vi "Set Write Access.vi"(8 "error in (no error)":errorcluster, 10 "Write Access":enum8{"Allowed", "Required", "None"}(ring), 11 "abs_SharedVar_Bool in":refnum<class "conc_SharedVar_DBL.lvclass">) -> (0 "error out":errorcluster, 3 "abs_SharedVar_Bool out":refnum<class "conc_SharedVar_DBL.lvclass">)   [LabVIEW 2021, in "conc_SharedVar_DBL.lvclass"]
uses:
  conc_SharedVar_DBL.lvclass
  conc_SharedVar_DBL.lvclass/conc_SharedVar_DBL.ctl
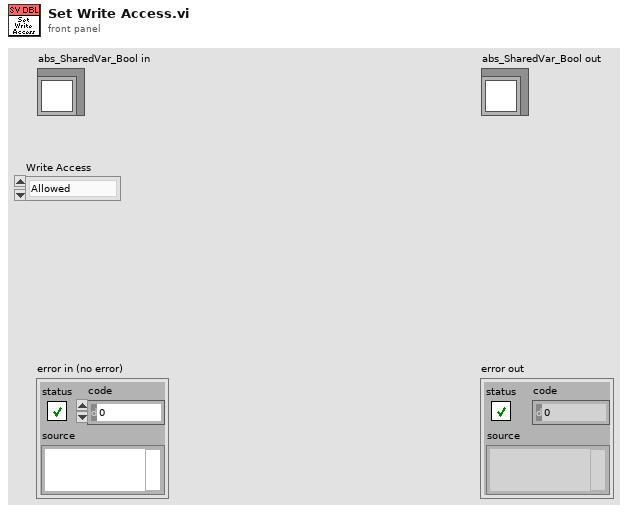
[diagram p1: front panel]
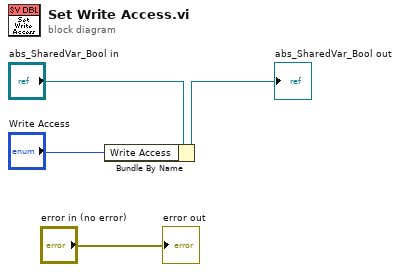
[diagram p0: block diagram]
diagram:
  n1 = Bundle By Name(cluster="abs_SharedVar_Bool in", "Write Access"="Write Access") -> (→"abs_SharedVar_Bool out":refnum<class "conc_SharedVar_DBL.lvclass">)
  "error out" <- "error in (no error)"
